vi "runTestScenario.vi"(8 "error in (no error)":errorcluster, 11 "Digital Input Test  in":refnum<class "Digital Input Test.lvclass">) -> (0 "error out":errorcluster, 1 "Result":T1, 2 "TestExecution":T2, 3 "Digital Input Test out":refnum<class "Digital Input Test.lvclass">)   [LabVIEW 2015, in "Digital Input Test.lvclass"]
uses:
  Digital Input Test.lvclass
  Typedefs/TestExecution.ctl
  Typedefs/PassFailTest.ctl
  Typedefs/WriteLogMessageInput.ctl
  Typedefs/TestScenarioTypes.ctl
  Typedefs/Digital Signal Level.ctl
  Digital Input Test.lvclass/Digital Input Test.ctl
  Model/TestLog/ITestLog/ITestLog.lvclass
  Model/ReadILCStrategy/IReadILCStrategy/IReadILCStrategy.lvclass
  Model/ConfigureILCStrategy/IConfigureILCStrategy/IConfigureILCStrategy.lvclass
  Typedefs/ILCBTTypedefs.lvlib
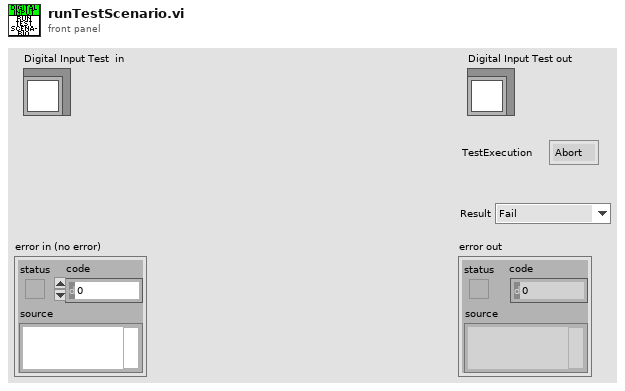
[diagram p1: front panel]
types:
  T1 = typedef "ILCBTTypedefs.lvlib/PassFailTest.ctl" = enum16{"Fail", "Pass", "NA"}
  T2 = typedef "ILCBTTypedefs.lvlib/TestExecution.ctl" = enum16{"Abort", "Continue"}
  T3 = typedef "ILCBTTypedefs.lvlib/Digital Signal Level.ctl" = enum16{"Low", "High"}
  T4 = typedef "ILCBTTypedefs.lvlib/WriteLogMessageInput.ctl" = cluster{"Test Scenario":T5, "Description":string, "Actual Value":string, "Data File":string, "Result":T1}
  T5 = typedef "ILCBTTypedefs.lvlib/TestScenarioTypes.ctl" = enum16{"+3.3VA Supply Test", "+3.3VD Supply Test", "+5VA Supply Test", "+5VD Supply Test", "Unique ID Test", "TEDS Status Test", "LIMSW1_TTL Low Test", "LIMSW1_TTL High Test", "LIMSW2_TTL Low Test", "LIMSW2_TTL High Test", "Tachometer Low Test", "Tachometer High Test", "SSR_TTL Low Test", "SSR_TTL High Test", "SM_GPI Low Test", "SM_GPI High Test", "CW Motion Without Limit Test", "CW Motion With Limit Test", "CW Motion With Both Limits Test", "CW Motion on CCW Limit Test", "CCW Motion Without Limit Test", "CCW Motion With Limit Test", "CCW Motion With Both Limits Test", "CCW Motion on CW Limit Test", "RS232-TXD Low Test", "RS232-TXD High Test", "RS232-RTS Low Test", "RS232-RTS High Test", "RS232-RXD Low Test", "RS232-RXD High Test", "RS232-CTS Low Test", "RS232-CTS High Test", "Out_SS Low Test", "Out_SS High Test", "Out_SDI Low Test", "Out_SDI High Test", "Out_SCLK Low Test", "Out_SCLK High Test", "Reset Low Test", "Reset High Test", "1 Channel ADC Test", "3 Channel ADC Test", "5 Channel ADC Test", "Vref Test", "ROT Test", "DAC1 Test", "DAC2 Test", "DAC3 Test", "DAC4 Test", "BIAS Test", "EXC1 Test", "EXC2 Test", "EXC3 Test", "EXC4 Test"}
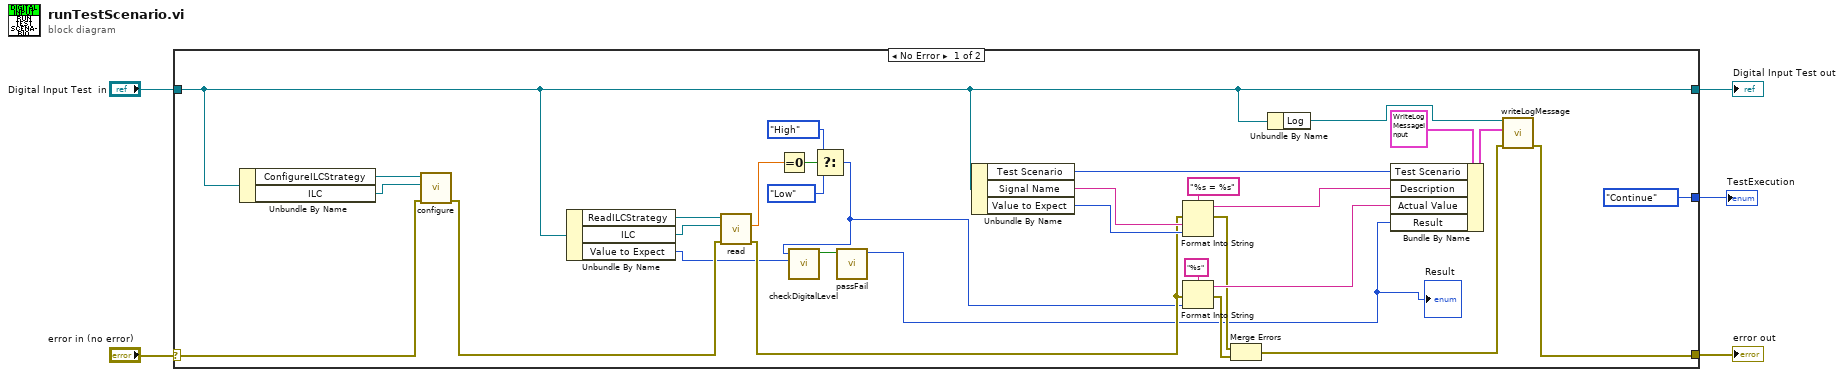
[diagram p0: block diagram]
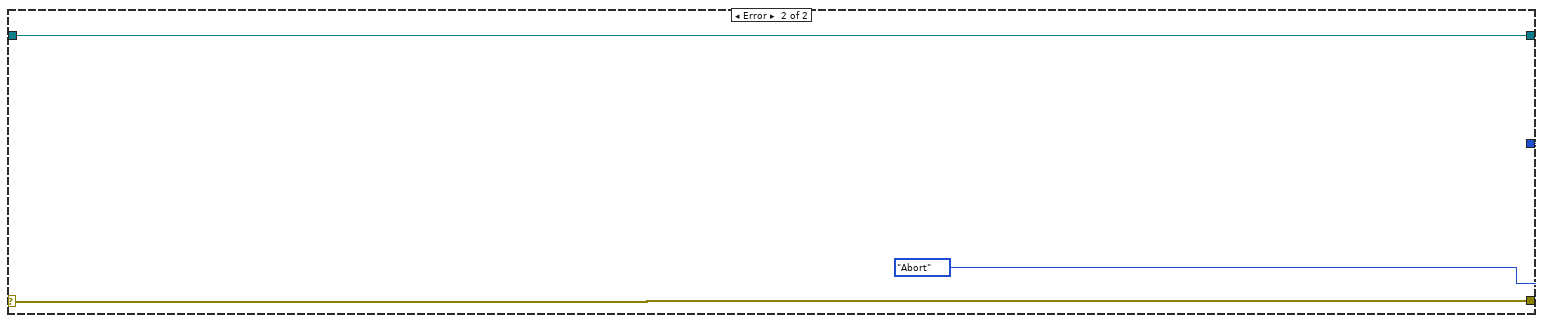
[diagram p2: hidden frame]
diagram:
  n1 = case shown="No Error" "error in (no error)" {
    selector: "error in (no error)" -> [w17 w39]
    tunnel: [w36 w39] -> w4
    tunnel: [TestExecution."Continue" ("TestExecution") TestExecution."Abort" ("TestExecution")] -> w3
    tunnel: "Digital Input Test  in" -> [w19 w37]
    tunnel: [w19 w37] -> w1
    frame No Error {
      n2 = Unbundle By Name(w19) -> ("ConfigureILCStrategy"=w33:refnum<class "IConfigureILCStrategy.lvclass">, "ILC"=w34:refnum<class "ILC.lvclass">)
      n3 = call-dynamic "configure.vi"("error in (no error)"=w17, "ILC"=w34, "IConfigureILCStrategy in"=w33) -> ("error out"=w14:errorcluster)  [unwired: 7 in, 1 out]
      n4 = Unbundle By Name(w19) -> ("ReadILCStrategy"=w16:refnum<class "IReadILCStrategy.lvclass">, "ILC"=w15:refnum<class "ILC.lvclass">, "Value to Expect"=w12:T3)
      n5 = call-dynamic "read.vi"("error in (no error)"=w14, "ILC"=w15, "IReadILCStrategy in"=w16) -> ("error out"=w13:errorcluster, "Value"=w11:dbl)  [unwired: 6 in, 1 out]
      n6 = Equal To 0?(x=w11) -> (x = 0?=w10:bool)
      n7 = Select(t=Digital_Signal_Level."High" ("Digital Signal Level"), s=w10, f=Digital_Signal_Level."Low" ("Digital Signal Level")) -> (s? t:f=w7:T3)
      n8 = call "checkDigitalLevel.vi"("Expected"=w12, "Actual"=w7) -> ("Pass?"=w32:bool)  [unwired: 9 in]
      n9 = call "passFail.vi"("Boolean"=w32) -> ("Result"=w6:T1)  [unwired: 10 in]
      "Result" <- w6
      n10 = Unbundle By Name(w19) -> ("Test Scenario"=w25:T5, "Signal Name"=w30:string, "Value to Expect"=w20:T3)
      n11 = Format Into String(format string="%s = %s", error in=w13, w30, w20) -> (resulting string=w26:string, error out=w23:errorcluster)  [unwired: 1 in]
      n12 = Format Into String(format string="%s", error in=w13, w7) -> (resulting string=w27:string, error out=w24:errorcluster)  [unwired: 1 in]
      n13 = Merge Errors(w23, w24) -> (w22:errorcluster)
      n14 = Unbundle By Name(w19) -> ("Log"=w18:refnum<class "ITestLog.lvclass">)
      n15 = Bundle By Name(cluster=T4 {"Test Scenario"=enum."+3.3VA Supply Test", "Description"="", "Actual Value"="", "Data File"="", "Result"=enum."Fail"} ("WriteLogMessageInput"), "Test Scenario"=w25, "Description"=w26, "Actual Value"=w27, "Result"=w6) -> (w28:T4)
      n16 = call-dynamic "writeLogMessage.vi"("error in (no error)"=w22, "WriteLogMessageInput"=w28, "ITestLog in"=w18) -> ("error out"=w36:errorcluster)  [unwired: 7 in, 1 out]
    }
    frame Error {
    }
  }
  "Digital Input Test out" <- w1
  "error out" <- w4
  "TestExecution" <- w3
